vi "Util_ConvertImageToLatest.vi"(8 "error in (no error)":errorcluster, 11 "Image Path":path) -> (0 "error out":errorcluster)   [LabVIEW 2023]
panel:
  in  "State Variables":cluster{"CurrentFile":path}
  in  "Cancel":bool
  in  "Start":bool
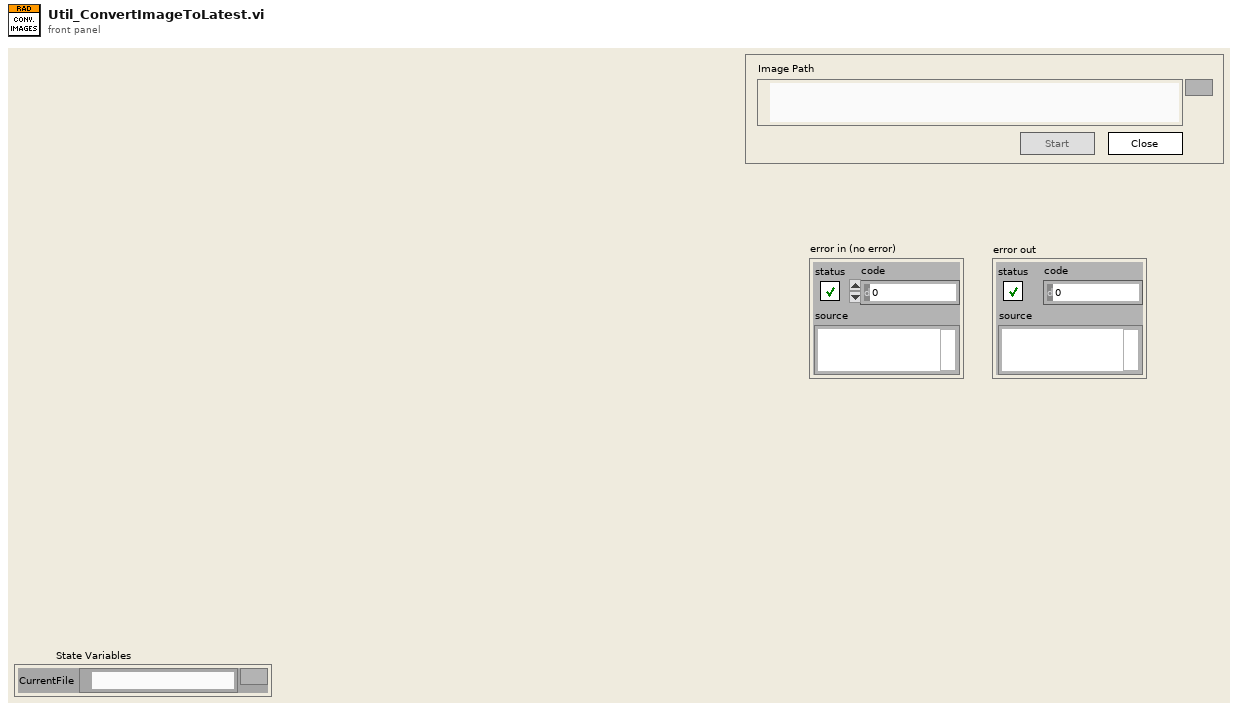
[diagram p1: front panel]
types:
  T1 = enum8{"Enabled", "Disabled", "Disabled and Grayed Out"}
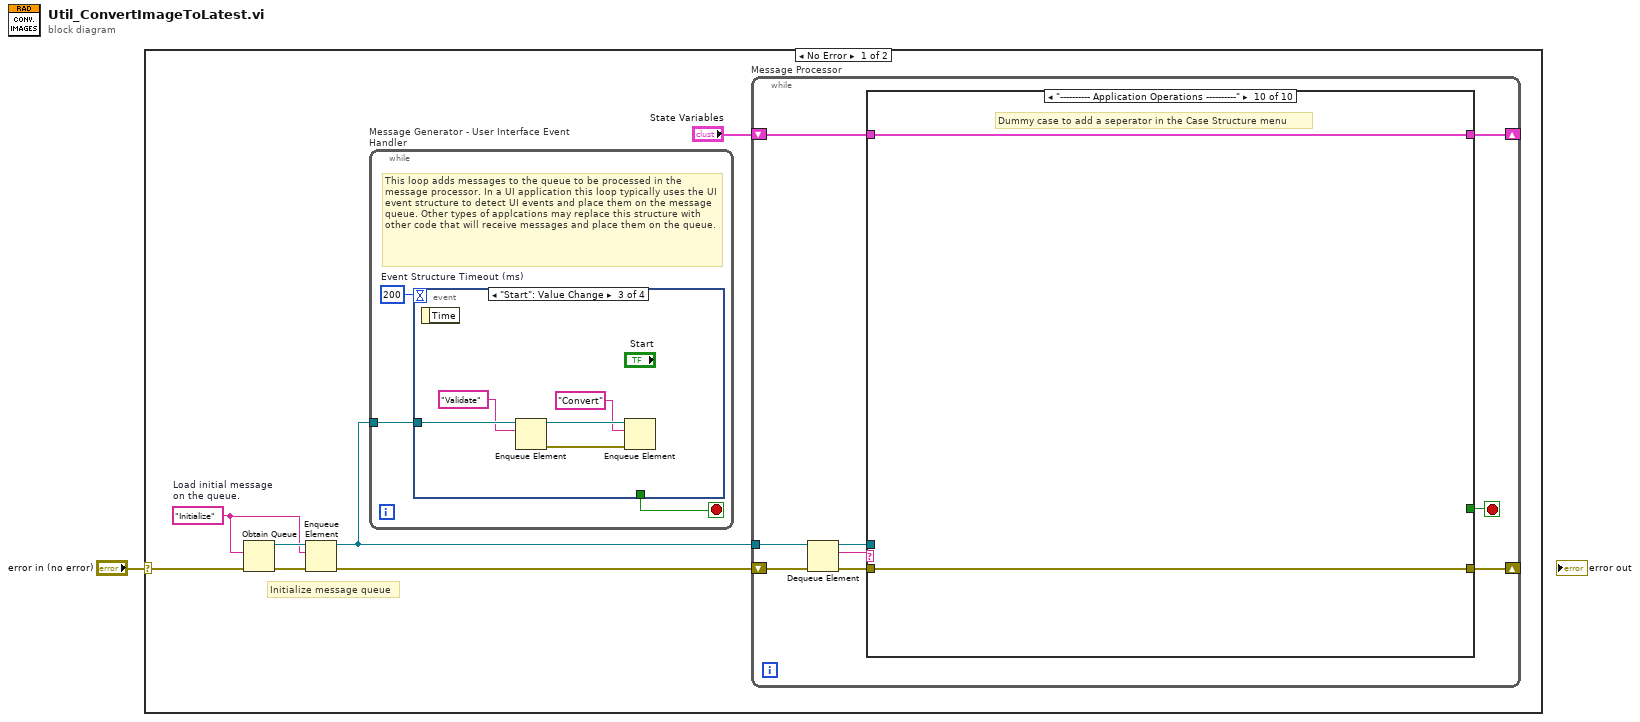
[diagram p0: block diagram]
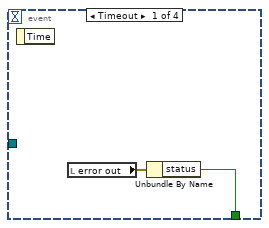
[diagram p2: hidden frame]
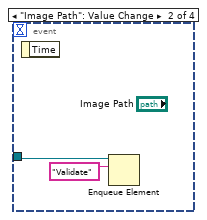
[diagram p3: hidden frame]
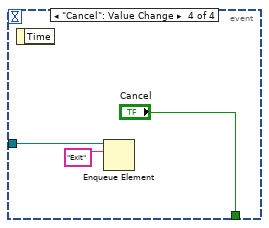
[diagram p4: hidden frame]
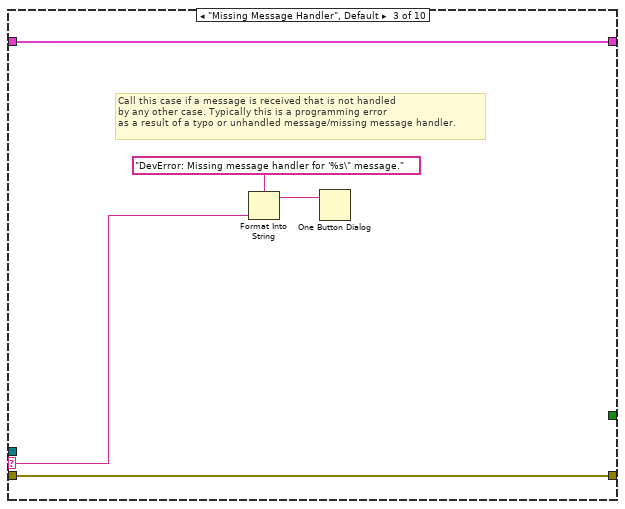
[diagram p7: hidden frame]
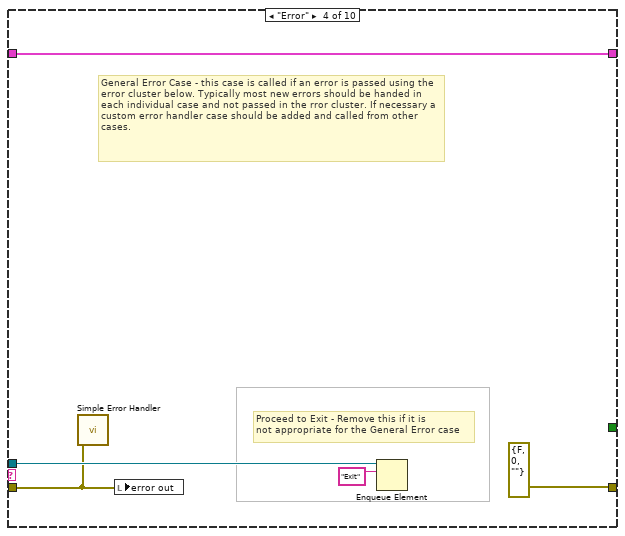
[diagram p8: hidden frame]
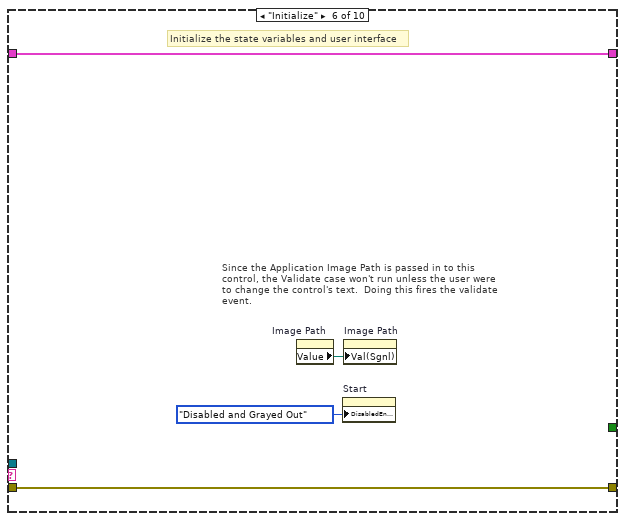
[diagram p10: hidden frame]
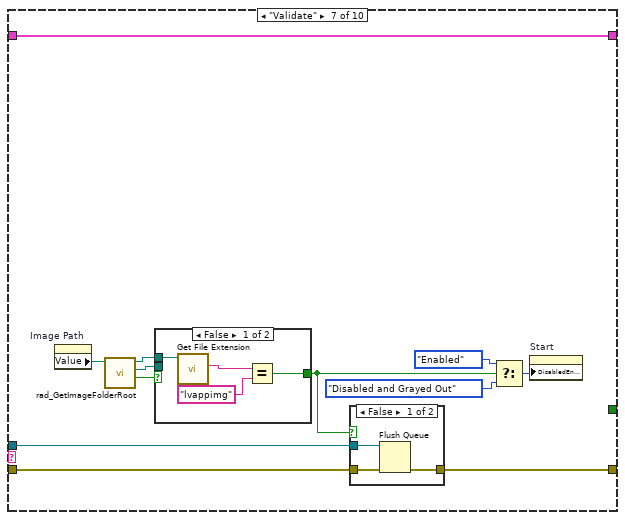
[diagram p11: hidden frame]
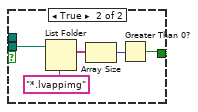
[diagram p13: hidden frame]
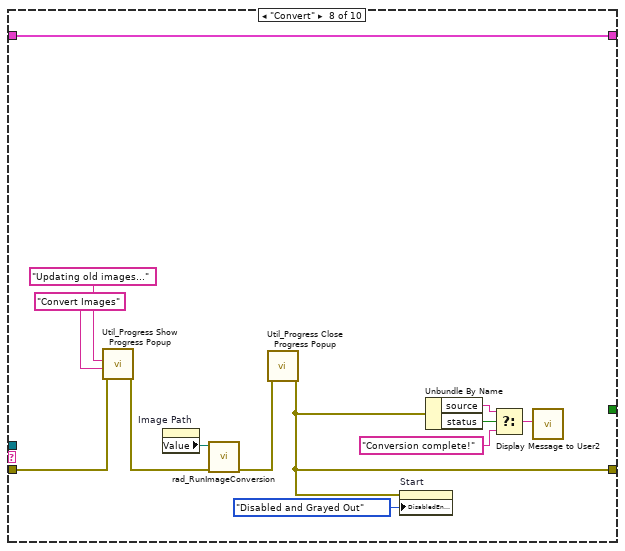
[diagram p14: hidden frame]
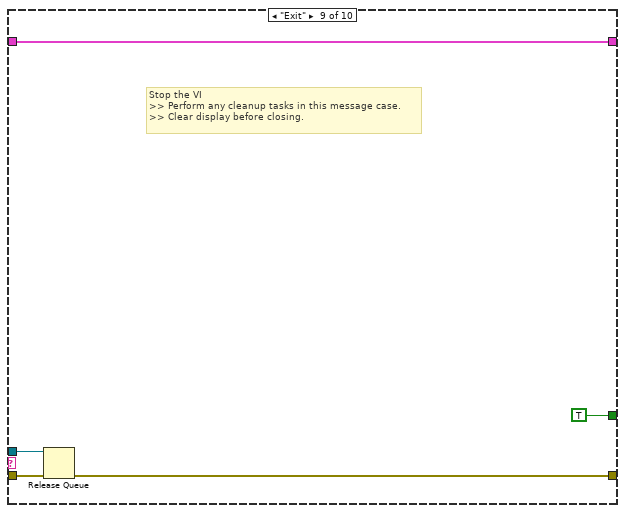
[diagram p15: hidden frame]
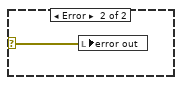
[diagram p16: hidden frame]
diagram:
  n1 = case shown="No Error" "error in (no error)" {
    selector: "error in (no error)" -> [w6 w98]
    frame No Error {
      w2 = "Initialize"  # Load initial message on the queue.
      # "Initialize message queue"
      n2 = Obtain Queue(element data type=w2, error in (no error)=w6) -> (queue out=w4:refnum<queue>, error out=w8:errorcluster)  [unwired: 3 in, 1 out]
      n3 = Enqueue Element(queue=w4, element=w2, error in (no error)=w8) -> (queue out=w3:refnum<queue>, error out=w5:errorcluster)  [unwired: 1 in, 1 out]
      n4 = while "Message Generator - User Interface Event Handler" {
        tunnel: w3 -> [w9]
        stop <- w10 stop-if-true
        w11 = 200  # Event Structure Timeout (ms)
        # "This loop adds messages to the queue to be processed in the message processor. In a UI application this loop typically uses the UI event structure to detect UI events and place them on the message queue. Other types of applcations may replace this structure with other code that will receive messages and place them on the queue."
        n5 = event shown="[2] \"Start\": Value Change" {
          selector: _ -> [_ _ _ _]
          dyn-events: _ -> [_ _ _ _]
          timeout: w11 -> [_ _ _ _]
          tunnel: [w12 _ _ "Cancel"] -> w10
          tunnel: w9 -> [_ w14 w20 w23]
          event Timeout {
            n6 = event-data() -> ()  [unwired: 2 out]
            n7 = local read "error out"() -> (w13:errorcluster)
            n8 = Unbundle By Name(w13) -> ("status"=w12:bool)
          }
          event "Image Path": Value Change {
            n9 = event-data() -> ()  [unwired: 2 out]
            n10 = Enqueue Element(queue=w14, element="Validate" ("Message Name")) -> ()  [unwired: 2 in, 3 out]
          }
          event "Start": Value Change {
            n11 = event-data() -> ()  [unwired: 2 out]
            n12 = Enqueue Element(queue=w20, element="Validate" ("Name")) -> (queue out=w19:refnum<queue>, error out=w16:errorcluster)  [unwired: 2 in, 1 out]
            n13 = Enqueue Element(queue=w19, element="Convert", error in (no error)=w16) -> ()  [unwired: 1 in, 3 out]
          }
          event "Cancel": Value Change {
            n14 = event-data() -> ()  [unwired: 2 out]
            n15 = Enqueue Element(queue=w23, element="Exit" ("Message Name")) -> ()  [unwired: 2 in, 3 out]
          }
        }
      }
      n16 = while "Message Processor" {
        shift-left: w5 -> [w27]
        shift-right: [w30] -> _
        tunnel: w3 -> [w28]
        shift-left: "State Variables" -> [w32]
        shift-right: [w31] -> _
        stop <- w24 stop-if-true
        n17 = Dequeue Element(queue=w28, error in (no error)=w27) -> (queue out=w29:refnum<queue>, element=w25:string, error out=w26:errorcluster)  [unwired: 1 in, 1 out]
        n18 = case shown="\"---------- Application Operations ----------\"" w25 {
          selector: w25 -> [_ _ w39 _ _ _ _ _ _ _]
          tunnel: [w34 w36 w41 w46 w48 w52 w64 w90 w95 w97] -> w31
          tunnel: w32 -> [w34 w36 w41 w46 w48 w52 w64 w90 w95 w97]
          tunnel: w29 -> [_ _ _ w44 _ _ w55 _ w93 _]
          tunnel: w26 -> [w33 w35 w40 w42 w47 w51 w54 w82 w94 w96]
          tunnel: [w33 w35 w40 errorcluster {"status"=FALSE, "code"=0, "source"=""} ("error out") w47 w51 w53 w79 w92 w96] -> w30
          tunnel: [_ _ _ _ _ _ _ _ TRUE _] -> w24
          frame "---------- Framework Operations ----------" {
            # "Dummy case to add a seperator in the Case Structure menu"
          }
          frame "", "Idle" {
            # "Idle Case - this case is called after a Timeout on the Get Next Message from Queue VI, if no new messages are present on the queue. This case can be used for housekeeping tasks such as updating the UI."
          }
          frame "Missing Message Handler", Default {
            # "Call this case if a message is received that is not handled \nby any other case. Typically this is a programming error\nas a result of a typo or unhandled message/missing message handler."
            n19 = Format Into String(format string="DevError: Missing message handler for '%s\" message." ("message"), w39) -> (resulting string=w37:string)  [unwired: 2 in, 1 out]
            n20 = One Button Dialog(message=w37) -> ()  [unwired: 2 out]
          }
          frame "Error" {
            # "Proceed to Exit - Remove this if it is\nnot appropriate for the General Error case"
            # "General Error Case - this case is called if an error is passed using the error cluster below. Typically most new errors should be handed in each individual case and not passed in the rror cluster. If necessary a custom error handler case should be added and called from other cases."
            n21 = call <vilib>:"Simple Error Handler.vi"("error in (no error)"=w42) -> ()  [unwired: 1 in, 8 out]
            n22 = local write "error out"(w42) -> ()
            n23 = Enqueue Element(queue=w44, element="Exit") -> ()  [unwired: 2 in, 3 out]
          }
          frame "---------- Generic Operations ----------" {
            # "Dummy case to add a seperator in the Case Structure menu"
          }
          frame "Initialize" {
            # "Since the Application Image Path is passed in to this\ncontrol, the Validate case won't run unless the user were\nto change the control's text.  Doing this fires the validate\nevent."
            # "Initialize the state variables and user interface"
            n24 = property on="Image Path" class="Path"() -> ("Value"=w49:path)  [unwired: 2 in, 2 out]
            n25 = property on="Start" class="Bool"("DisabledEnum"=T1."Disabled and Grayed Out" ("Disabled")) -> ()  [unwired: 2 in, 2 out]
            n26 = property on="Image Path" class="Path"("Val(Sgnl)"=w49) -> ()  [unwired: 2 in, 2 out]
          }
          frame "Validate" {
            n27 = property on="Image Path" class="Path"() -> ("Value"=w63:path)  [unwired: 2 in, 2 out]
            n28 = call "rad_GetImageFolderRoot.vi"("Image Path"=w63) -> ("directory"=w62:bool, "ImageFolderRoot"=w61:path, "Image Path out"=w60:path)  [unwired: 3 in, 1 out]
            n29 = case shown="False" w62 {
              tunnel: w61 -> [_ w76]
              tunnel: w60 -> [w72 _]
              tunnel: [w69 w73] -> w56
              frame False {
                n30 = call <vilib>:"Get File Extension.vi"("file"=w72) -> ("lowercase file extension"=w71:string)  [unwired: 6 in, 4 out]
                n31 = Equal?(x=w71, y="lvappimg") -> (x = y?=w69:bool)
              }
              frame True {
                n32 = List Folder(path=w76, pattern="*.lvappimg") -> (filenames=w75:string[])  [unwired: 2 in, 3 out]
                n33 = Array Size(array=w75) -> (size(s)=w74:i32)
                n34 = Greater Than 0?(x=w74) -> (x > 0?=w73:bool)
              }
            }
            n35 = case shown="False" w56 {
              tunnel: w55 -> [w67 _]
              tunnel: w54 -> [w66 w68]
              tunnel: [w65 w68] -> w53
              frame False {
                n36 = Flush Queue(queue=w67, error in (no error)=w66) -> (error out=w65:errorcluster)  [unwired: 2 out]
              }
              frame True {
              }
            }
            n37 = Select(t=T1."Enabled" ("Disabled"), s=w56, f=T1."Disabled and Grayed Out") -> (s? t:f=w57:T1)
            n38 = property on="Start" class="Bool"("DisabledEnum"=w57) -> ()  [unwired: 2 in, 2 out]
          }
          frame "Convert" {
            n39 = call "Util_Progress Show Progress Popup.vi"("error in (no error)"=w82, "Title"="Convert Images", "Message"="Updating old images...") -> ("error out"=w81:errorcluster)  [unwired: 8 in]
            n40 = property on="Image Path" class="Path"() -> ("Value"=w85:path)  [unwired: 2 in, 2 out]
            n41 = call "rad_RunImageConversion.vi"("error in"=w81, "Image Path"=w85) -> ("error out"=w80:errorcluster)  [unwired: 5 in]
            n42 = call "Util_Progress Close Progress Popup.vi"("error in (no error)"=w80) -> ("error out"=w79:errorcluster)  [unwired: 10 in]
            n43 = property on="Start" class="Bool"(error in=w79, "DisabledEnum"=T1."Disabled and Grayed Out" ("Disabled")) -> ()  [unwired: 1 in, 2 out]
            n44 = Unbundle By Name(w79) -> ("source"=w88:string, "status"=w89:bool)
            n45 = Select(t=w88, s=w89, f="Conversion complete!") -> (s? t:f=w87:string)
            n46 = call "Display Message to User2"("Message"=w87) -> ()  [unwired: 9 in, 2 out]
          }
          frame "Exit" {
            # "Stop the VI\n>> Perform any cleanup tasks in this message case.\n>> Clear display before closing."
            n47 = Release Queue(queue=w93, error in (no error)=w94) -> (error out=w92:errorcluster)  [unwired: 1 in, 2 out]
          }
          frame "---------- Application Operations ----------" {
            # "Dummy case to add a seperator in the Case Structure menu"
          }
        }
      }
    }
    frame Error {
      n48 = local write "error out"(w98) -> ()
    }
  }
